vi "DriverStation Game Data.vi"() -> (3 "Game Specific Data":string)   [LabVIEW 2026, in "MrcLib.lvlib"]
doc: "Returns game specific data from the FMS (Field Management System)."
uses:
  MrcLib.lvlib
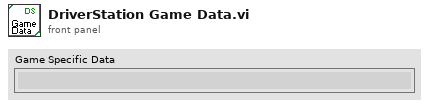
[diagram p1: front panel]
types:
  T1 = typedef "MrcLib.lvlib/MRC_ControlData.ctl" = cluster{"controlFlags":u32, "matchTime":u16, "currentOpMode":u64, "gameDataLength":u8, "gameData":cluster{"gameData 0":u8, "gameData 1":u8, "gameData 2":u8, "gameData 3":u8, "gameData 4":u8, "gameData 5":u8, "gameData 6":u8, "gameData 7":u8}}
  T2 = cluster{"gameData 0":u8, "gameData 1":u8, "gameData 2":u8, "gameData 3":u8, "gameData 4":u8, "gameData 5":u8, "gameData 6":u8, "gameData 7":u8}
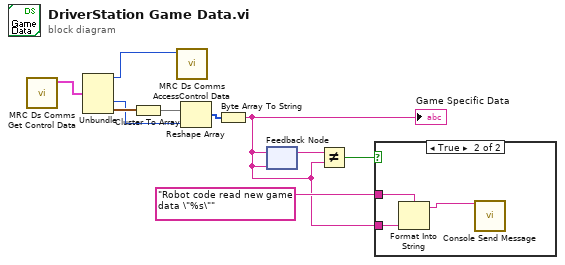
[diagram p0: block diagram]
diagram:
  n1 = call "MRC Ds Comms Get Control Data.vi"() -> ("data out"=w7:T1)  [unwired: 10 in, 1 out]
  n2 = Unbundle(w7) -> ("controlFlags"=w1:u32, "gameDataLength"=w3:u8, "gameData"=w4:T2)  [unwired: 2 out]
  n3 = Cluster To Array(cluster=w4) -> (array=w6:u8[])
  n4 = call "MRC Ds Comms AccessControl Data.vi"("controlFlag"=w1) -> ()  [unwired: 7 in, 4 out]
  n5 = Reshape Array(w6, w3) -> (w5:u8[])
  n6 = Byte Array To String(unsigned byte array=w5) -> (string=w2:string)
  "Game Specific Data" <- w2
  n7 = feedback #1(w2) -> (w10:string)
  n8 = feedback-in #1(w2) -> ()
  n9 = Not Equal?(x=w10, y=w2) -> (x != y?=w9:bool)
  n10 = case shown="True" w9 {
    tunnel: "Robot code read new game data \"%s\"" ("Message") -> [_ w13]
    tunnel: w2 -> [_ w12]
    frame False {
    }
    frame True {
      n11 = Format Into String(format string=w13, w12) -> (resulting string=w11:string)  [unwired: 2 in, 1 out]
      n12 = call "Console Send Message.vi"("Message"=w11) -> ()  [unwired: 14 in, 1 out]
    }
  }
